vi "DataSort.vi"(4 "Runs":u32[](array[numeric]), 6 "PXI":dbl[][][](array[numeric]), 7 "PXI i":i32[][](array[numeric]), 8 "eDAQ":dbl[][][](array[numeric]), 9 "eDAQ i":i32[][](array[numeric]), 10 "cDAQ":dbl[][](array[numeric]), 11 "cDAQ i":i32[](array[numeric])) -> (3 "Data Out":dbl[][](array[numeric]))   [LabVIEW 2013]
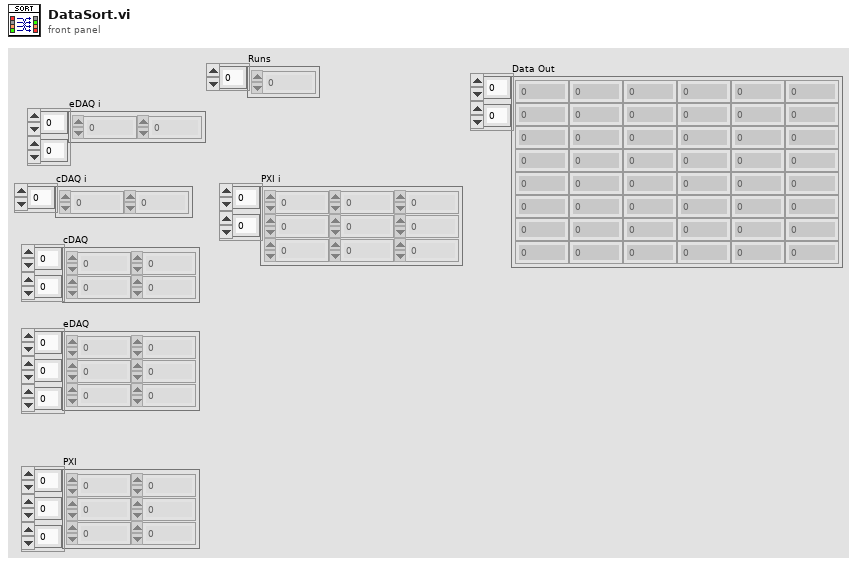
[diagram p1: front panel]
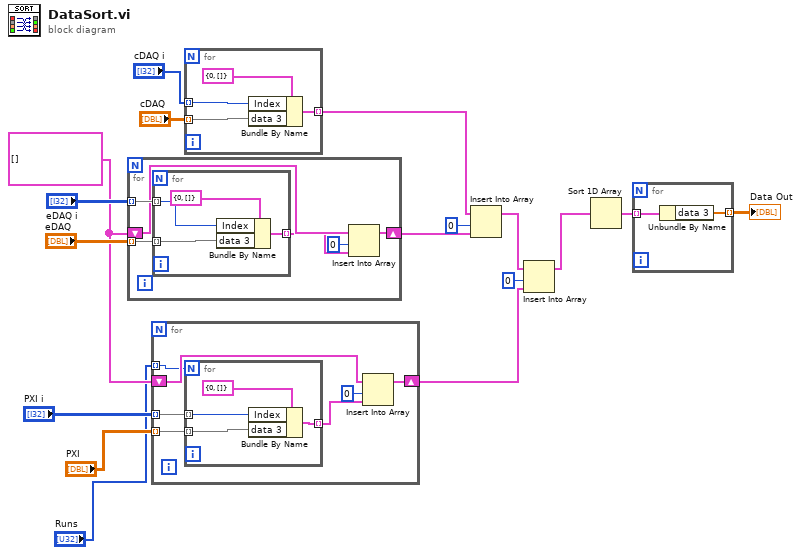
[diagram p0: block diagram]
diagram:
  w7 = cluster{"Index":i32, "data 3":dbl[]}[] []
  n1 = for {
    tunnel: "eDAQ" -> [w23] mode=indexing
    tunnel: "eDAQ i" -> [w22] mode=indexing
    shift-right: [w19] -> w13
    shift-left: w7 -> [w21]
    n2 = for {
      tunnel: w22 -> [w26] mode=indexing
      tunnel: w23 -> [w25] mode=indexing
      tunnel: [w24] -> w20 mode=indexing
      n3 = Bundle By Name(cluster=cluster{"Index":i32, "data 3":dbl[]} {"Index"=0, "data 3"=[]}, "Index"=w26, "data 3"=w25) -> (w24:cluster{"Index":i32, "data 3":dbl[]})
    }
    n4 = Insert Into Array(array=w21, index=0, new element=w20) -> (w19:cluster{"Index":i32, "data 3":dbl[]}[])
  }
  n5 = for {
    tunnel: "PXI i" -> [w34] mode=indexing
    tunnel: "PXI" -> [w29] mode=indexing
    shift-right: [w33] -> w3
    shift-left: w7 -> [w32]
    tunnel: "Runs" -> [w28] mode=indexing
    n6 = for {
      N: w28 -> [_]
      tunnel: w34 -> [w37] mode=indexing
      tunnel: w29 -> [w36] mode=indexing
      tunnel: [w35] -> w31 mode=indexing
      n7 = Bundle By Name(cluster=cluster{"Index":i32, "data 3":dbl[]} {"Index"=0, "data 3"=[]}, "Index"=w37, "data 3"=w36) -> (w35:cluster{"Index":i32, "data 3":dbl[]})
    }
    n8 = Insert Into Array(array=w32, index=0, new element=w31) -> (w33:cluster{"Index":i32, "data 3":dbl[]}[])
  }
  n9 = for {
    tunnel: "cDAQ i" -> [w41] mode=indexing
    tunnel: "cDAQ" -> [w40] mode=indexing
    tunnel: [w39] -> w14 mode=indexing
    n10 = Bundle By Name(cluster=cluster{"Index":i32, "data 3":dbl[]} {"Index"=0, "data 3"=[]}, "Index"=w41, "data 3"=w40) -> (w39:cluster{"Index":i32, "data 3":dbl[]})
  }
  n11 = Insert Into Array(array=w14, index=0, new element=w13) -> (w6:cluster{"Index":i32, "data 3":dbl[]}[])
  n12 = Insert Into Array(array=w6, index=0, new element=w3) -> (w5:cluster{"Index":i32, "data 3":dbl[]}[])
  n13 = Sort 1D Array(array=w5) -> (sorted array=w12:cluster{"Index":i32, "data 3":dbl[]}[])
  n14 = for {
    tunnel: w12 -> [w44] mode=indexing
    tunnel: [w43] -> w11 mode=indexing
    n15 = Unbundle By Name(w44) -> ("data 3"=w43:dbl[])
  }
  "Data Out" <- w11
